vi "Main.vi"() -> ()   [LabVIEW 2022 SP3, in "VideoMux.lvlib"]
uses:
  VideoMux.lvlib
  VideoMux/VideoMux.lvclass
panel:
  out "error out":errorcluster
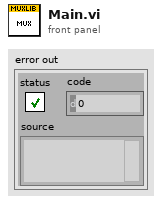
[diagram p1: front panel]
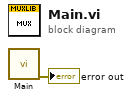
[diagram p0: block diagram]
diagram:
  n1 = call "Main.vi"() -> ("error out"=→"error out":errorcluster)  [unwired: 11 in]
